vi "get_setpoint.vi"(8 "error in (no error)":errorcluster, 10 "channel":dbl, 11 "Lakeshore_336 in":refnum<class "Lakeshore_336.lvclass">) -> (0 "error out":errorcluster, 2 "setpoint":string, 3 "Lakeshore_336 out":refnum<class "Lakeshore_336.lvclass">)   [LabVIEW 2018, in "Lakeshore_336.lvclass"]
doc: "reads the setpoint of the \"channel\" from the actual instrument"
uses:
  Lakeshore_336.lvclass
  instrument.lvclass
  Drivers/Lake Shore 336/Lake Shore 336.lvlib
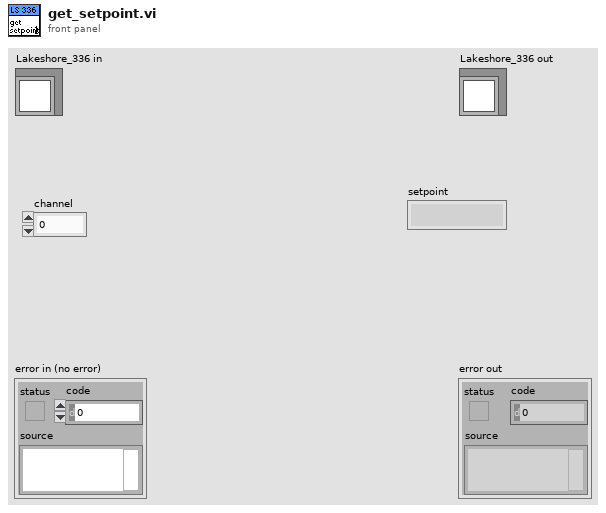
[diagram p1: front panel]
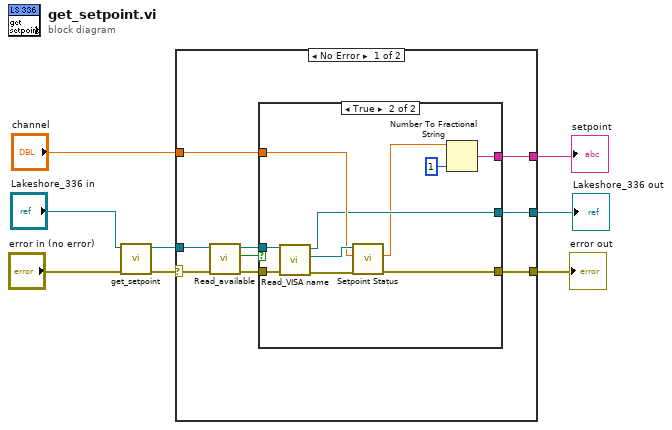
[diagram p0: block diagram]
diagram:
  n1 = call-parent "get_setpoint.vi"("error in (no error)"="error in (no error)", "instrument in"="Lakeshore_336 in") -> ("error out"=w6:errorcluster, "instrument out"=w5:refnum<class "Lakeshore_336.lvclass">)  [unwired: 7 in, 1 out]
  n2 = case shown="No Error" w6 {
    selector: w6 -> [w12 w31]
    tunnel: w5 -> [w13 w30]
    tunnel: "channel" -> [w17 _]
    tunnel: [w16 w31] -> w3
    tunnel: [w15 w30] -> w2
    tunnel: [w14 _] -> w1
    frame No Error {
      n3 = call-dynamic "Read_available.vi"("error in (no error)"=w12, "instrument in"=w13) -> ("error out"=w10:errorcluster, "available?"=w9:bool, "instrument out"=w11:refnum<class "Lakeshore_336.lvclass">)  [unwired: 7 in]
      n4 = case shown="True" w9 {
        tunnel: w17 -> [_ w27]
        tunnel: [w18 w26] -> w16
        tunnel: [w19 w25] -> w15
        tunnel: [_ w23] -> w14
        tunnel: w11 -> [w19 w21]
        tunnel: w10 -> [w18 w20]
        frame False {
        }
        frame True {
          n5 = call-dynamic "Read_VISA name.vi"("error in (no error)"=w20, "instrument in"=w21) -> ("error out"=w28:errorcluster, "VISA resource name"=w29:refnum<visa-resource-name>, "instrument out"=w25:refnum<class "Lakeshore_336.lvclass">)  [unwired: 7 in]
          n6 = call "Setpoint Status.vi"("error in (no error)"=w28, "Output (1:1)"=w27, "VISA resource name"=w29) -> ("error out"=w26:errorcluster, "Setpoint"=w24:dbl)  [unwired: 6 in, 1 out]
          n7 = Number To Fractional String(number=w24, precision (6)=i16 1) -> (F-format string=w23:string)  [unwired: 2 in]
        }
      }
    }
    frame Error {
    }
  }
  "error out" <- w3
  "Lakeshore_336 out" <- w2
  "setpoint" <- w1
